vi "Save Load Accuracy Data(2).vi"(8 "error in (no error)":errorcluster, 10 "AD Counts":dbl[][](array[numeric]), 11 "Accuracy Loads":dbl[][](array[numeric])) -> (0 "error out":errorcluster, 2 "Error Code":i32, 3 "Pass?":bool)   [LabVIEW 2013]
uses:
  <vilib>/Utility/NIReport.llb/NI_report.lvclass
  <vilib>/addons/_office/excel.llb/Excel Easy Table (num).vi
  <vilib>/addons/_office/NI_ReportGenerationToolkit.lvlib
  <vilib>/Utility/NIReport.llb/Excel/NI_Excel.lvclass
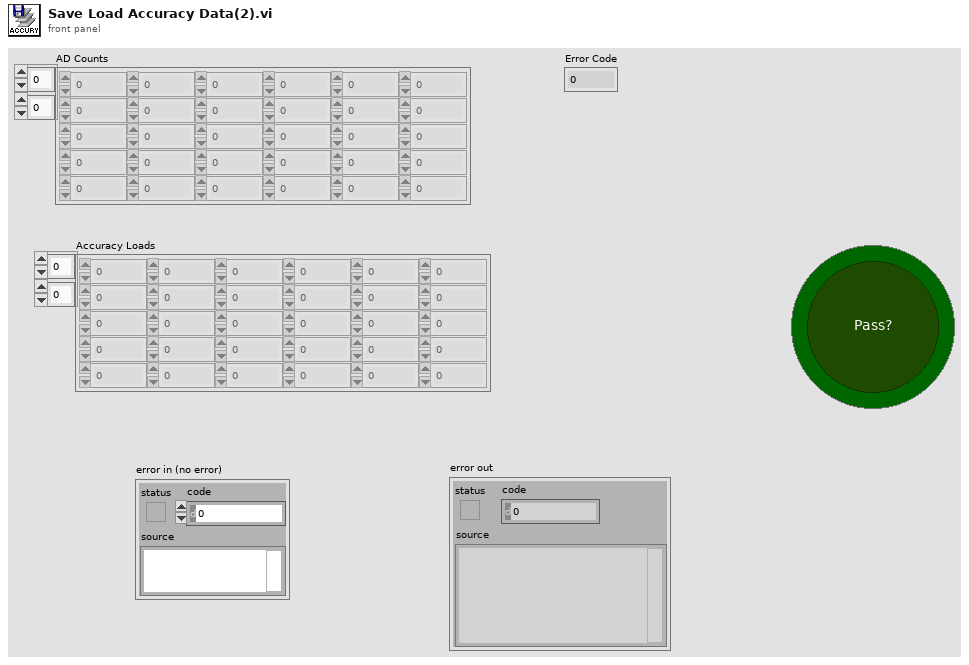
[diagram p1: front panel]
types:
  T1 = enum16{"maximized", "minimized", "normal", "no change"}
  T2 = enum16{"Standard Report", "HTML", "Word", "Excel"}
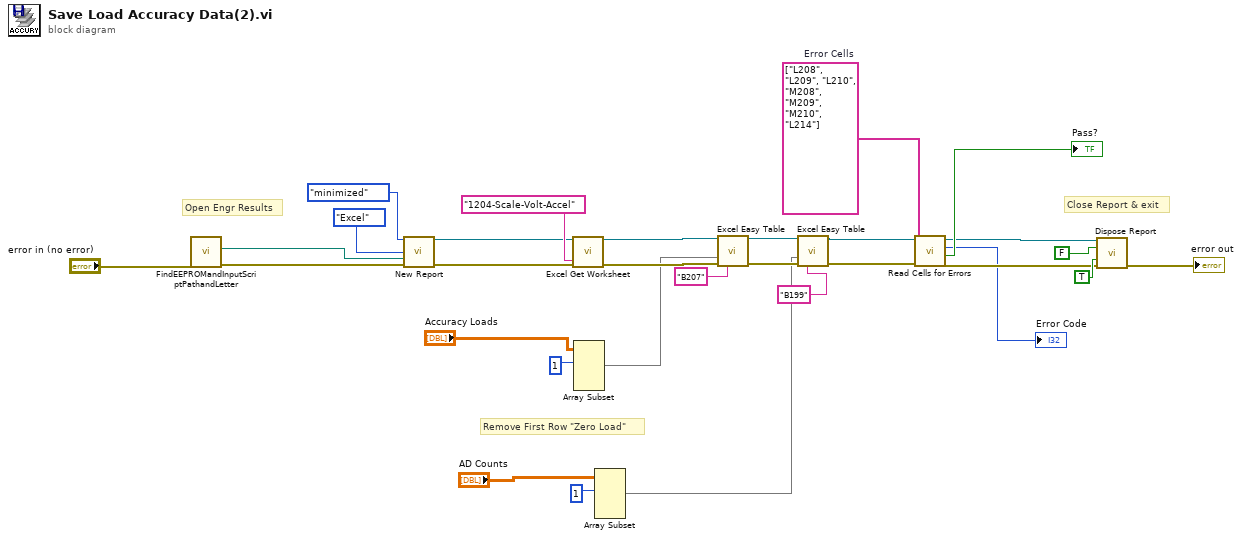
[diagram p0: block diagram]
diagram:
  w12 = string[] ["L208", "L209", "L210", "M208", "M209", "M210", "L214"]  # Error Cells
  # "Remove First Row \"Zero Load\""
  # "Close Report & exit"
  # "Open Engr Results"
  n1 = call "FindEEPROMandInputScriptPathandLetter.vi"("Error In"="error in (no error)") -> ("Error Out"=w21:errorcluster, "Engr Result Path"=w30:path)  [unwired: 6 in, 1 out]
  n2 = call <vilib>:"New Report.vi"("window state (normal)"=T1."minimized", "report type"=T2."Excel", "template (empty)"=w30, "error in (no error)"=w21) -> ("report out"=w24:refnum<class "NI_report.lvclass">, "error out"=w23:errorcluster)  [unwired: 10 in]
  n3 = call <vilib>:"Excel Get Worksheet.vi"("report in"=w24, "error in (no error)"=w23, "name (\"\")"="1204-Scale-Volt-Accel" ("name (\"\")")) -> ("report out"=w20:refnum<class "NI_report.lvclass">, "error out"=w19:errorcluster)  [unwired: 11 in]
  n4 = Array Subset(array="Accuracy Loads", index (row)=1 ("length")) -> (w9:dbl[][])  [unwired: 3 in]
  n5 = Array Subset(array="AD Counts", index (row)=1 ("length")) -> (w2:dbl[][])  [unwired: 3 in]
  n6 = call-poly <vilib>:"Excel Easy Table.vi"("report in"=w20, "text data"=w9, "error in (no error)"=w19, "name (\"\")"="B207" ("name (\"\")")) -> ("report out"=w6:refnum<class "NI_report.lvclass">, "error out"=w5:errorcluster)  [unwired: 7 in, 3 out]
  n7 = call-poly <vilib>:"Excel Easy Table.vi"("report in"=w6, "text data"=w2, "error in (no error)"=w5, "name (\"\")"="B199" ("name (\"\")")) -> ("report out"=w4:refnum<class "NI_report.lvclass">, "error out"=w3:errorcluster)  [unwired: 7 in, 3 out]
  n8 = call "Read Cells for Errors.vi"("error in (no error)"=w3, "Error Cells (ex:A12)"=w12, "NI_report in"=w4) -> ("error out"=w16:errorcluster, "Pass?"=→"Pass?":bool, "Error Code"=→"Error Code":i32, "NI_report out"=w17:refnum<class "NI_report.lvclass">)  [unwired: 5 in]
  n9 = call-dynamic "Dispose Report.vi"("report in"=w17, "wait until printing completed? (T)"=FALSE, "save changes? (F)"=TRUE, "error in (no error)"=w16) -> ("error out"=→"error out":errorcluster)  [unwired: 11 in]
